vi "Configure Session.vi"(8 "error in":errorcluster, 11 "Plugin in":refnum<class "Adjust Block Size.lvclass">) -> (0 "error out":errorcluster, 3 "Plugin out":refnum<class "Adjust Block Size.lvclass">)   [LabVIEW 2024, in "Adjust Block Size.lvlib" / "Adjust Block Size.lvclass"]
uses:
  Adjust Block Size.lvclass
  C:/Program Files/National Instruments/LabVIEW 2024/vi.lib/FlexLogger/SDK/PluginSDK.lvlibp/PEFClasses/SDK/Plugin/Plugin.lvclass
  Adjust Block Size.lvclass/Adjust Block Size.ctl
  <vilib>/FlexLogger/SDK/PluginSDK.lvlibp/PEFClasses/SDK/Producer Channel/Producer Channel.lvclass
  C:/Program Files/National Instruments/LabVIEW 2024/vi.lib/FlexLogger/SDK/PluginSDK.lvlibp/PEFClasses/SDK/Channel/Channel.lvclass
  <vilib>/FlexLogger/SDK/PluginSDK.lvlibp/PEFClasses/SDK/Plugin/ParameterAccess/Read DBL.vi
  <vilib>/FlexLogger/SDK/PluginSDK.lvlibp/PEFClasses/SDK/Plugin/ParameterAccess/Read N Channel.vi
  <vilib>/FlexLogger/SDK/PluginSDK.lvlibp/PEFClasses/SDK/Producer Channel/Create Producer Channel_v2.vi
  <vilib>/FlexLogger/SDK/PluginSDK.lvlibp/PEFClasses/SDK/Plugin/Get Valid Producer Channels.vi
  <vilib>/FlexLogger/SDK/PluginSDK.lvlibp/PEFClasses/SDK/Plugin/Plugin.lvclass
  <vilib>/addons/_NISVFA/_Shared subVIs/Data Objects/Waveforms (DBL)/Waveforms (N Ch).lvclass
  <vilib>/FlexLogger/SDK/PluginSDK.lvlibp
  C:/Program Files/National Instruments/LabVIEW 2024/vi.lib/FlexLogger/SDK/PluginSDK.lvlibp/PEFClasses/SDK/Processing Element/Processing Element.lvclass
  C:/dev/dsb/niflexlogger-plugins/PDK plugins/Adjust Block Size/Adjust Block Size.lvclass
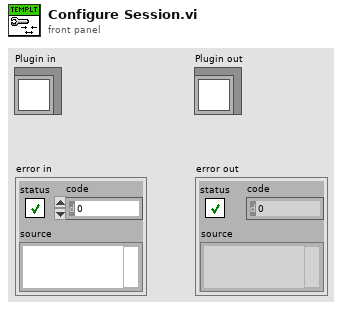
[diagram p1: front panel]
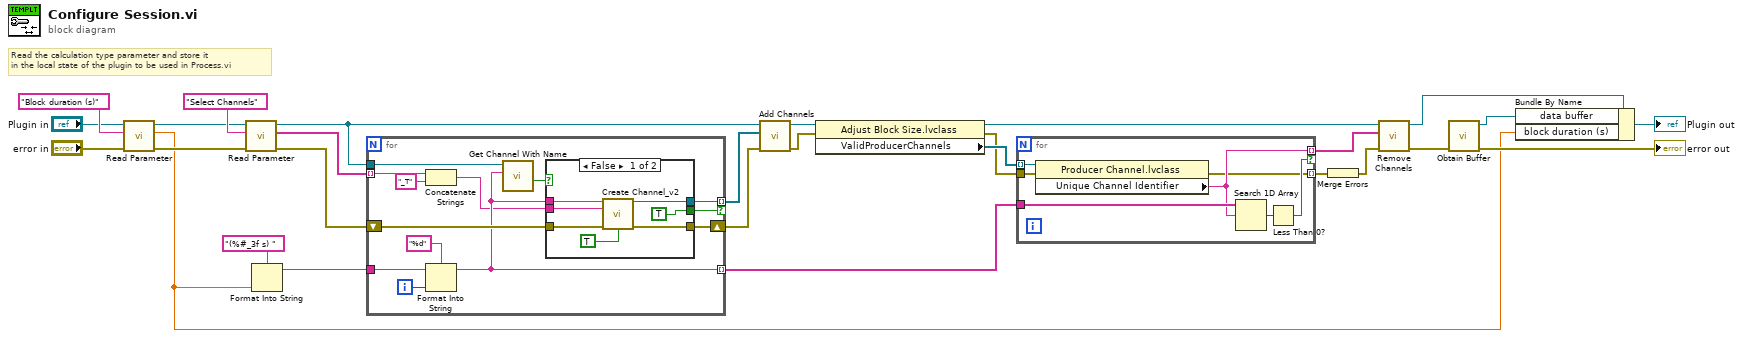
[diagram p0: block diagram]
diagram:
  # "Read the calculation type parameter and store it\nin the local state of the plugin to be used in Process.vi"
  n1 = call-poly <vilib>:"Read Parameter.vi"("error in (no error)"="error in", "Name"="Block duration (s)", "Plugin in"="Plugin in") -> ("error out"=w17:errorcluster, "Value"=w6:dbl, "Plugin out"=w19:refnum<class "Adjust Block Size.lvclass">)  [unwired: 5 in, 1 out]
  n2 = call-poly <vilib>:"Read Parameter.vi"("error in (no error)"=w17, "Name (Unique Channel Identifier)"="Select Channels" ("Name"), "Plugin in"=w19) -> ("error out"=w23:errorcluster, "Channels"=w21:string[], "Plugin out"=w15:refnum<class "Adjust Block Size.lvclass">)  [unwired: 5 in, 1 out]
  n3 = Format Into String(format string="(%#_3f s) ", w6) -> (resulting string=w4:string)  [unwired: 2 in, 1 out]
  n4 = for {
    shift-right: [w41] -> w24
    shift-left: w23 -> [w40]
    tunnel: [w39] -> w22 mode=indexing if=w34
    tunnel: w21 -> [w32] mode=indexing
    tunnel: w15 -> [w36]
    tunnel: [w33] -> w11 mode=indexing
    tunnel: w4 -> [w31]
    i -> [w37]
    n5 = Concatenate Strings(w32, "_T" ("string")) -> (w30:string)
    n6 = Format Into String(format string="%d", initial string=w31, w37) -> (resulting string=w33:string)  [unwired: 1 in, 1 out]
    n7 = call <vilib>:"Get Channel With Name.vi"("Name"=w33, "Plugin in"=w36) -> ("Found?"=w35:bool)  [unwired: 7 in, 2 out]
    n8 = case shown="False" w35 {
      tunnel: [w48 w49] -> w41
      tunnel: w40 -> [w46 w49]
      tunnel: [w45 _] -> w39
      tunnel: w33 -> [w44 _]
      tunnel: [TRUE ("Can Disable?") _] -> w34
      tunnel: w30 -> [w42 _]
      frame False {
        n9 = call-poly <vilib>:"Create Channel_v2.vi"("Unique Channel Identifier"=w44, "Default Channel Name"=w42, "error in (no error)"=w46, "Can Disable?"=TRUE) -> ("Producer Channel"=w45:refnum<class "Producer Channel.lvclass">, "error out"=w48:errorcluster)  [unwired: 10 in]
      }
      frame True {
      }
    }
  }
  n10 = call <vilib>:"Add Channels.vi"("error in (no error)"=w24, "Channels"=w22, "Plugin in"=w15) -> ("error out"=w13:errorcluster, "Plugin out"=w14:refnum<class "Adjust Block Size.lvclass">)  [unwired: 7 in]
  n11 = property class="Adjust Block Size.lvclass"(reference=w14, error in=w13) -> (reference out=w12:refnum<class "Adjust Block Size.lvclass">, error out=w3:errorcluster, "ValidProducerChannels"=w16:refnum<class "Producer Channel.lvclass">[])
  n12 = for {
    tunnel: w16 -> [w56] mode=indexing
    tunnel: [w54] -> w7 mode=indexing if=w52
    tunnel: w11 -> [w55]
    tunnel: w3 -> [w51]
    tunnel: [w50] -> w2 mode=indexing
    n13 = property class="Producer Channel.lvclass"(reference=w56, error in=w51) -> (error out=w50:errorcluster, "Unique Channel Identifier"=w54:string)  [unwired: 1 out]
    n14 = Search 1D Array(1D array=w55, element=w54) -> (index of element=w53:i32)  [unwired: 1 in]
    n15 = Less Than 0?(x=w53) -> (x < 0?=w52:bool)
  }
  n16 = Merge Errors(w2) -> (w1:errorcluster)
  n17 = call-dynamic "Remove Channels.vi"("error in (no error)"=w1, "Unique Channel Identifiers to Delete"=w7, "Plugin in"=w12) -> ("error out"=w8:errorcluster, "Plugin out"=w10:refnum<class "Adjust Block Size.lvclass">)  [unwired: 7 in]
  n18 = call <vilib>:"Obtain Buffer.vi"("error in (no error)"=w8) -> ("error out"=→"error out":errorcluster, "buffer out"=w26:refnum<data-value>)  [unwired: 9 in]
  n19 = Bundle By Name(cluster=w10, "data buffer"=w26, "block duration (s)"=w6) -> (→"Plugin out":refnum<class "Adjust Block Size.lvclass">)
